vi "H036 Harsh Pandit SCADA Lab 8a Sem 6.vi"() -> ()   [LabVIEW 2018]
panel:
  out "Concatenated String Length 2":i32
  out "Concatenated string":string
  out "String 2 Length":i32
  out "String 1 Length":i32
  in  "String 2":string
  in  "String 1":string
  # "Experoment 8A: Create a VI which consists of 2 string inputs. Find the length of each string\ninput. Display the combined string. Also find the length of combined string"
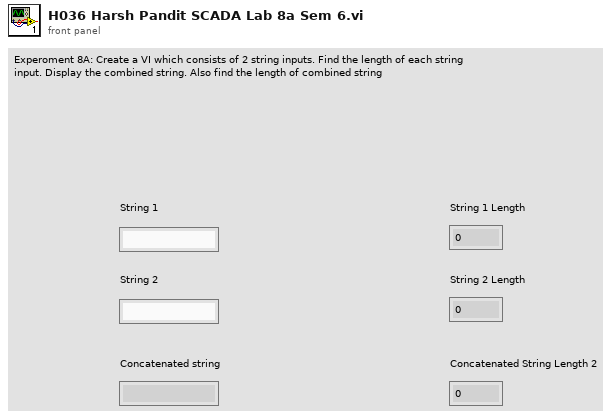
[diagram p1: front panel]
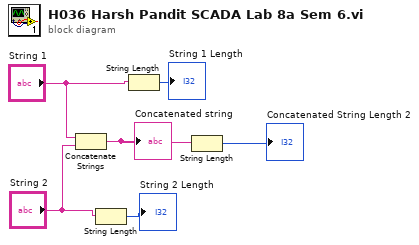
[diagram p0: block diagram]
diagram:
  n1 = Concatenate Strings("String 1", "String 2") -> (w1:string)
  "Concatenated string" <- w1
  n2 = String Length(string="String 2") -> (length=→"String 2 Length":i32)
  n3 = String Length(string="String 1") -> (length=→"String 1 Length":i32)
  n4 = String Length(string=w1) -> (length=→"Concatenated String Length 2":i32)
